vi "CG test stand thermocouple calibration and read.vi"() -> ()   [LabVIEW 2020]
doc: "This example demonstrates how to read N channels of analog input from a LINX device."
uses:
  <vilib>/MakerHub/LINX/Public/Peripherals/Analog/Analog Read N Chans.vi
  <vilib>/MakerHub/LINX/Private/Local IO/LinxAnalogRead.vi
  <vilib>/MakerHub/LINX/Public/Utilities/Check Channel.vi
  <vilib>/MakerHub/LINX/Public/Utilities/Open Serial.vi
  <vilib>/MakerHub/LINX/Private/Utilties/Generate Error.vi
  <vilib>/Analysis/Matrix/Numeric/Conversions/Array To Matrix - RA.vi
  <vilib>/Utility/file.llb/Write Delimited Spreadsheet (DBL).vi
  <vilib>/MakerHub/LINX/LMH-LINX.lvlib
  <vilib>/Analysis/Matrix/NI_Matrix.lvlib
panel:
  out "WRITING TO FILE":bool
  in  "?":bool
  out "error out":errorcluster
  out "Full filepath":string
  in  "Path":path
  in  "File extension":string
  in  "Filename":string
  in  "Analog Port":dbl
  out "Time Stamp":timestamp
  out "Input data":dbl(graph)
  out "Voltage":dbl
  in  "Stop Button":bool
  out "Loop Rate (Hz)":u32
  in  "Serial Port":refnum<visa-resource-name>
  # "X"
  # "+"
  # "CG test stand analog read\n\nThis VI works to read one single voltage value from an Arduino. Currently configured for a Mega 2560."
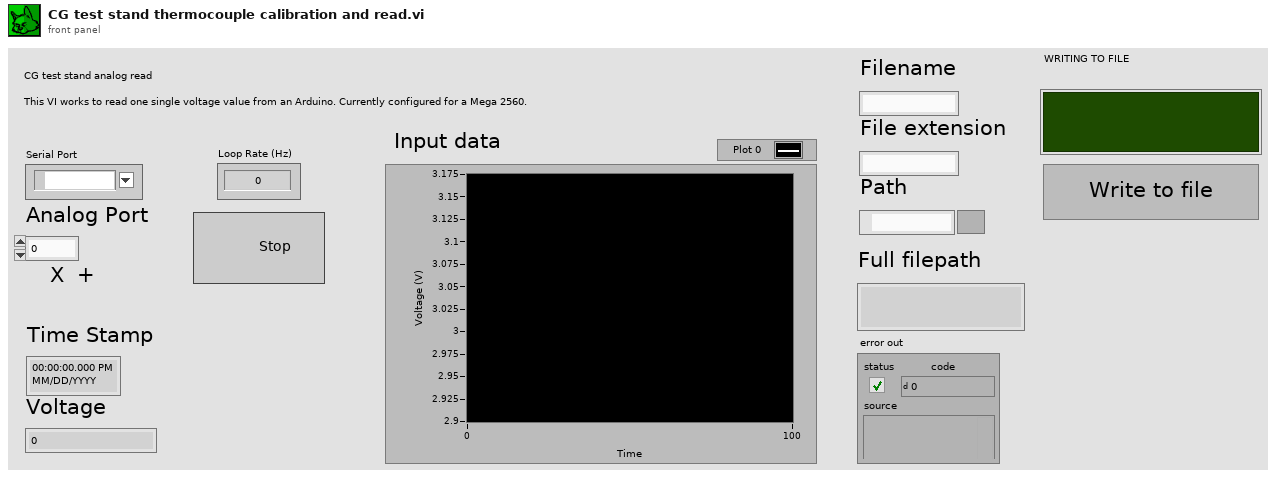
[diagram p1: front panel]
types:
  T1 = typedef "LMH-LINX.lvlib/LINX Ref.ctl" = cluster{"IO":T2, "Interface":T3, "LINX Device Config":T4}
  T2 = typedef "LMH-LINX.lvlib/Platform.ctl" = enum16{"Remote", "Local"}
  T3 = typedef "LMH-LINX.lvlib/Interface.ctl" = enum16{"Serial", "TCP"}
  T4 = typedef "LMH-LINX.lvlib/Device.lvlib/LINX Device Config.ctl" = cluster{"Interface":T3, "COM Port":refnum<visa-resource-name>, "TCP Configuration":T5, "Device Family":u8, "Device ID":u8, "Device Name":string, "TCP Ref":refnum<k5>, "Channels":T6}
  T5 = typedef "LMH-LINX.lvlib/Device.lvlib/TCP Config.ctl" = cluster{"IP Address":string, "Port":u16}
  T6 = typedef "LMH-LINX.lvlib/Channels.ctl" = cluster{"DI":u8[], "DO":u8[], "AI":u8[], "AO":u8[], "PWM":u8[], "QE":u8[], "UART":u8[], "I2C 2":u8[], "SPI":u8[], "CAN":u8[], "Servo":u8[], "AI Ref (V)":dbl, "AI Resolution (Bits)":u8, "AO Ref (V)":dbl, "AO Resolution (Bits)":u8}
  T7 = typedef "NI_Matrix.lvlib/RealMatrix.ctl" = dbl[][]
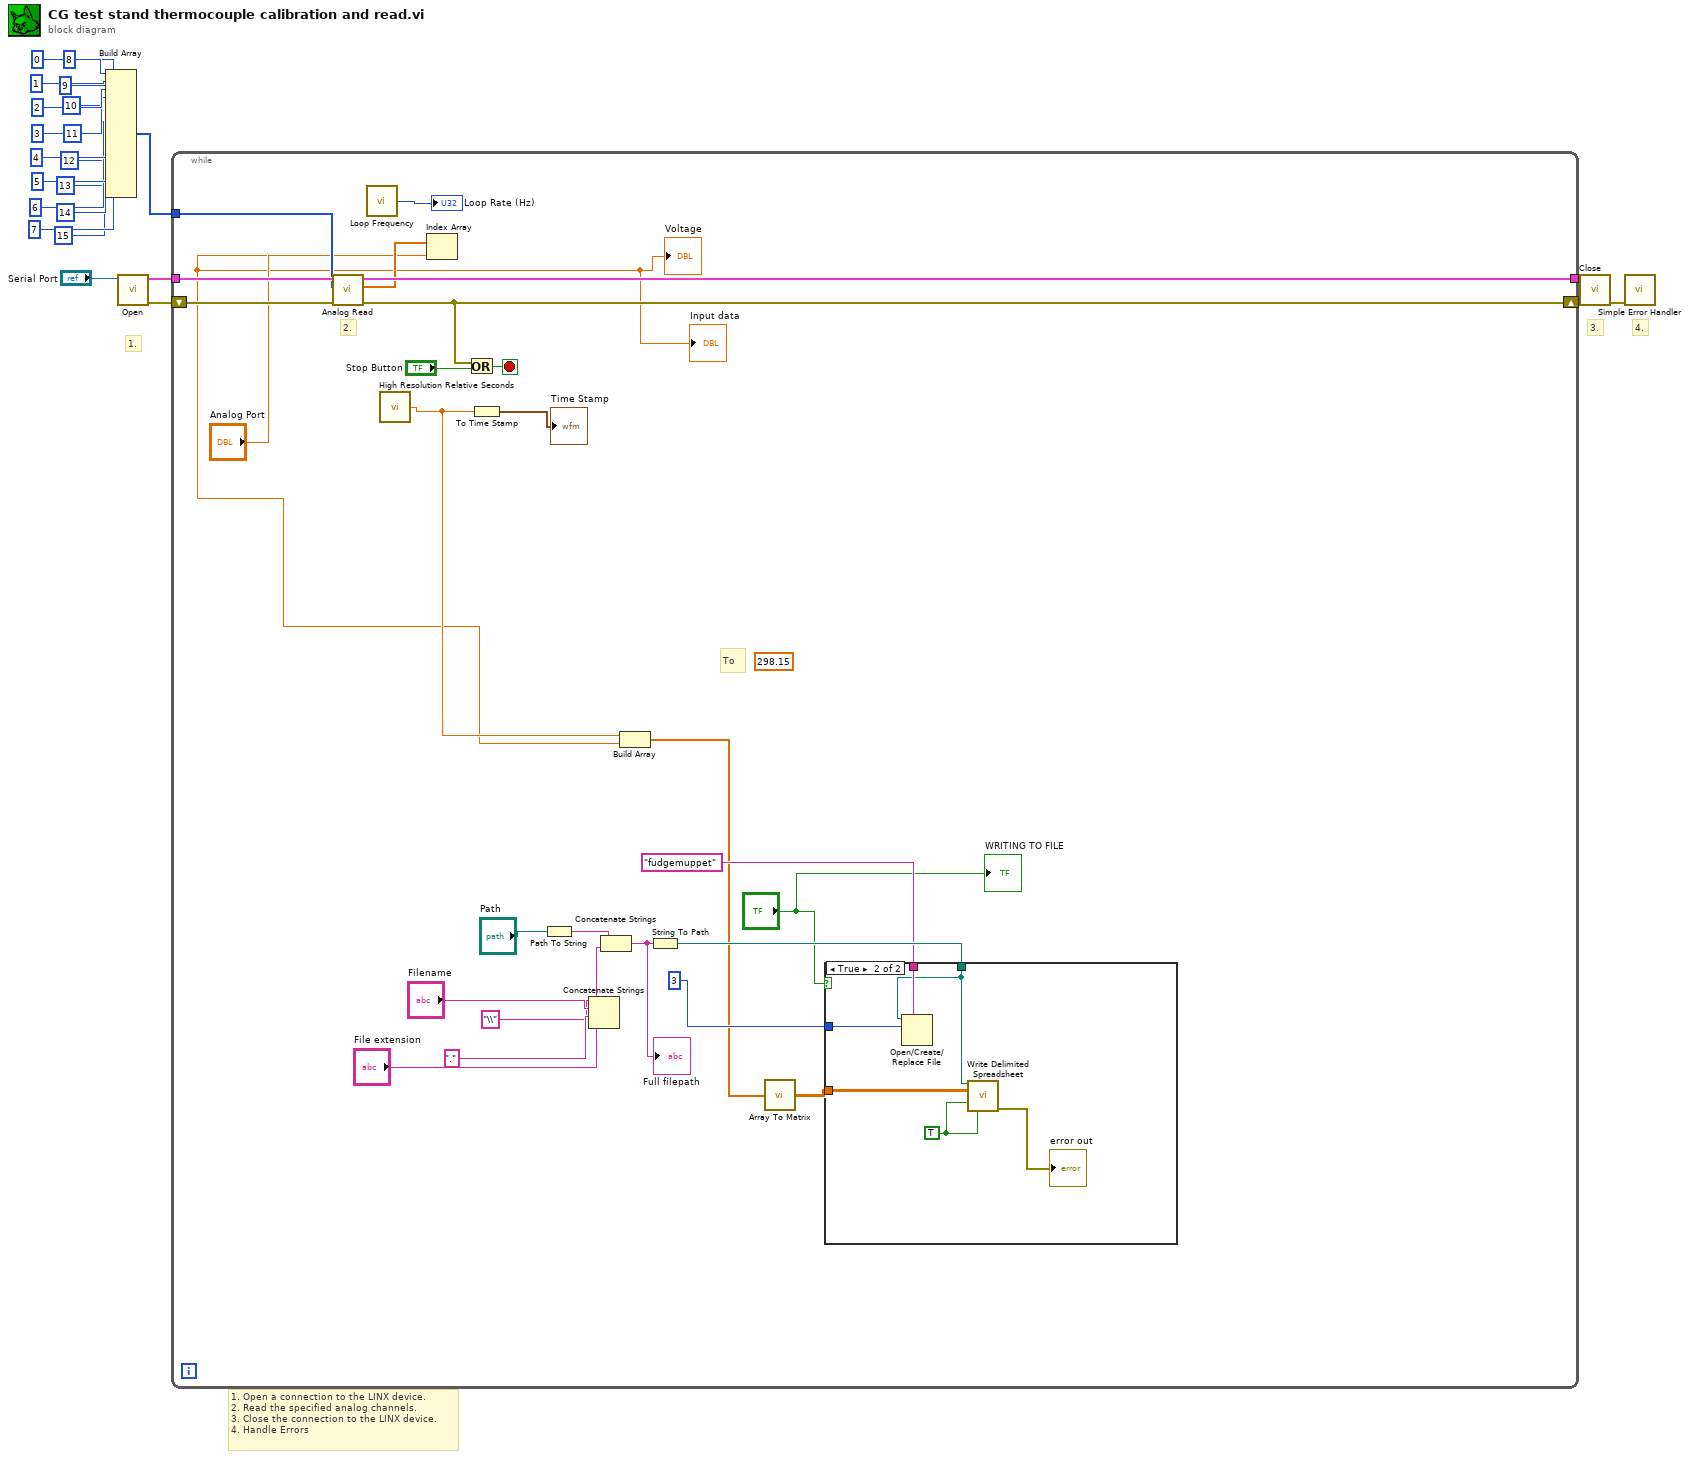
[diagram p0: block diagram]
diagram:
  # "1. Open a connection to the LINX device.\n2. Read the specified analog channels.\n3. Close the connection to the LINX device.\n4. Handle Errors"
  # "4."
  # "3."
  # "1."
  n1 = Build Array(0, 1, 2, 3, 4, 5, 6, 7, 8, 9, 10, 11, 12, 13, 14, 15) -> (w17:i32[])
  n2 = call-poly <vilib>:"Open.vi"("Serial Port"="Serial Port") -> ("Error Out"=w22:errorcluster, "LINX Resource"=w23:T1)  [unwired: 8 in, 1 out]
  n3 = while {
    tunnel: w23 -> [w50]
    tunnel: [w48] -> w21
    shift-right: [w45] -> w20
    shift-left: w22 -> [w49]
    tunnel: w17 -> [w44]
    stop <- w47 stop-if-true
    (unwired) 298.15
    # "To"
    # "2."
    n4 = call-poly <vilib>:"Analog Read.vi"("Error In"=w49, "AI Channel(s)"=w44, "LINX Resource"=w50) -> ("Error Out"=w45:errorcluster, "Voltages"=w43:dbl[], "LINX Resource"=w48:T1)  [unwired: 5 in, 1 out]
    n5 = call <vilib>:"Loop Frequency.vi"() -> ("Loop Rate (Hz)"=→"Loop Rate (Hz)":u32)
    n6 = call <vilib>:"High Resolution Relative Seconds.vi"() -> ("relative seconds"=w25:dbl)
    n7 = Index Array(array=w43, index="Analog Port") -> (element=w24:dbl)
    "Voltage" <- w24
    "Input data" <- w24
    n8 = Or(x=w45, y="Stop Button") -> (x .or. y?=w47:bool)
    n9 = To Time Stamp(1:w25) -> (0:→"Time Stamp":timestamp)
    n10 = Path To String(path="Path") -> (string=w38:string)
    n11 = Concatenate Strings("\\", "Filename", ".", "File extension") -> (w37:string)
    n12 = Concatenate Strings(w38, w37) -> (w36:string)
    "Full filepath" <- w36
    n13 = Build Array(w25, w24) -> (w26:dbl[])
    n14 = String To Path(string=w36) -> (path=w31:path)
    n15 = call-poly <vilib>:"Array To Matrix.vi"("Real 1D Array"=w26) -> ("Real Matrix (Column Vector)"=w27:T7)
    n16 = case shown="True" "?" {
      tunnel: w31 -> [_ w54]
      tunnel: w27 -> [_ w51]
      tunnel: "fudgemuppet" -> [_ w56]
      tunnel: 3 -> [_ w55]
      frame False {
      }
      frame True {
        w52 = TRUE
        n17 = Open/Create/Replace File(file path (use dialog)=w54, prompt=w56, operation (0:open)=w55) -> ()  [unwired: 3 in, 3 out]
        n18 = call-poly <vilib>:"Write Delimited Spreadsheet.vi"("file path (dialog if empty)"=w54, "2D data"=w51, "append to file? (new file:F)"=w52, "transpose? (no:F)"=w52) -> ("error out"=→"error out":errorcluster)  [unwired: 10 in, 1 out]
      }
    }
    "WRITING TO FILE" <- "?"
  }
  n19 = call <vilib>:"Close.vi"("Error In"=w20, "LINX Resource"=w21) -> ("Error Out"=w18:errorcluster)  [unwired: 9 in]
  n20 = call <vilib>:"Simple Error Handler.vi"("error in (no error)"=w18) -> ()  [unwired: 4 in, 5 out]
